vi "ControlPosition.vi"(6 "error in":errorcluster, 9 "Control in":refnum<class "Control.lvclass">) -> (0 "error out":errorcluster, 3 "Control out":refnum<class "Control.lvclass">, 5 "Position":T1)   [LabVIEW 2014, in "Control.lvclass"]
uses:
  Control.lvclass
  <vilib>/Utility/miscctls.llb/LVPositionTypeDef.ctl
  GObject/GObject.lvclass/GObject.ctl
  GObject/GObject.lvclass
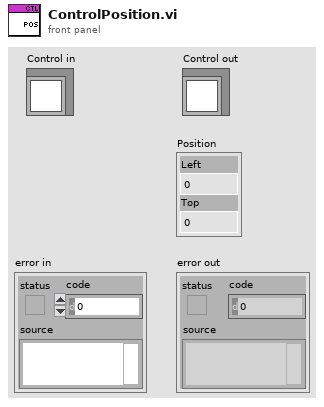
[diagram p1: front panel]
types:
  T1 = typedef "LVPositionTypeDef.ctl" = cluster{"Left":i32, "Top":i32}
  T2 = typedef "LVRectTypeDef.ctl" = cluster{"Left":i16, "Top":i16, "Right":i16, "Bottom":i16}
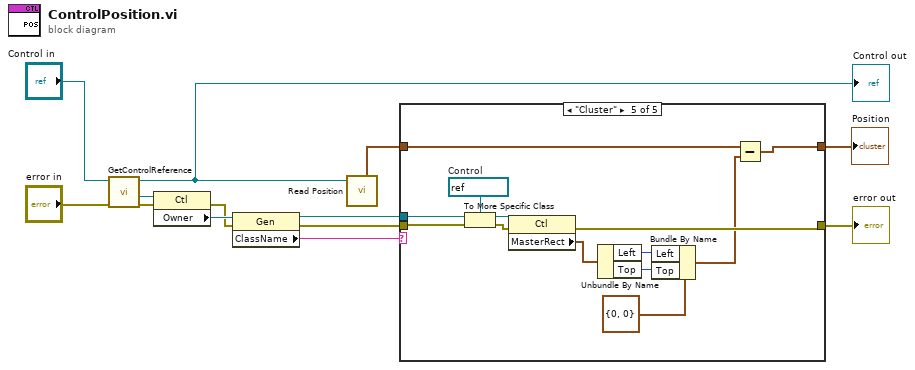
[diagram p0: block diagram]
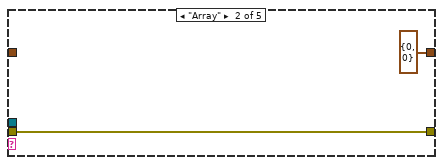
[diagram p3: hidden frame]
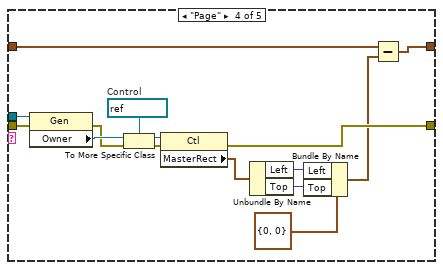
[diagram p5: hidden frame]
diagram:
  n1 = call "GetControlReference.vi"("error in"="error in", "Control in"="Control in") -> ("error out"=w10:errorcluster, "control reference"=w11:refnum<vi>, "Control out"=w2:refnum<class "Control.lvclass">)  [unwired: 7 in]
  "Control out" <- w2
  n2 = property class="Ctl"(reference=w11, error in=w10) -> (error out=w8:errorcluster, "Owner"=w9:refnum<vi>)  [unwired: 1 out]
  n3 = property class="Gen"(reference=w9, error in=w8) -> (reference out=w6:refnum<vi>, error out=w1:errorcluster, "ClassName"=w7:string)
  n4 = call "Read Position.vi"("GObject in"=w2) -> ("Position"=w5:T1)  [unwired: 7 in, 1 out]
  n5 = case shown="\"Cluster\"" w7 {
    tunnel: [w14 w17 w18 w25 w36] -> w3
    tunnel: w6 -> [_ _ _ w34 w44]
    tunnel: w5 -> [w15 _ w19 w30 w46]
    tunnel: [w15 T1 {"Left"=0, "Top"=0} ("Position") w19 w29 w45] -> w4
    tunnel: w1 -> [w14 w17 w18 w28 w43]
    frame Default {
    }
    frame "Array" {
    }
    frame "Panel" {
    }
    frame "Page" {
      w33 = refnum<vi> refnum  # Control
      n6 = property class="Gen"(reference=w34, error in=w28) -> (error out=w31:errorcluster, "Owner"=w32:refnum<vi>)  [unwired: 1 out]
      n7 = To More Specific Class(target class=w33, reference=w32, error in=w31) -> (specific class reference=w27:refnum<vi>, error out=w26:errorcluster)
      n8 = property class="Ctl"(reference=w27, error in=w26) -> (error out=w25:errorcluster, "MasterRect"=w24:T2)  [unwired: 1 out]
      n9 = Unbundle By Name(w24) -> ("Left"=w23:i16, "Top"=w22:i16)
      n10 = Bundle By Name(cluster=T1 {"Left"=0, "Top"=0} ("Position"), "Left"=w23, "Top"=w22) -> (w21:T1)
      n11 = Subtract(x=w30, y=w21) -> (x-y=w29:T1)
    }
    frame "Cluster" {
      w47 = refnum<vi> refnum  # Control
      n12 = To More Specific Class(target class=w47, reference=w44, error in=w43) -> (specific class reference=w38:refnum<vi>, error out=w37:errorcluster)
      n13 = property class="Ctl"(reference=w38, error in=w37) -> (error out=w36:errorcluster, "MasterRect"=w42:T2)  [unwired: 1 out]
      n14 = Unbundle By Name(w42) -> ("Left"=w41:i16, "Top"=w40:i16)
      n15 = Bundle By Name(cluster=T1 {"Left"=0, "Top"=0} ("Position"), "Left"=w41, "Top"=w40) -> (w35:T1)
      n16 = Subtract(x=w46, y=w35) -> (x-y=w45:T1)
    }
  }
  "error out" <- w3
  "Position" <- w4
